vi "Initialize-user-events.vi"(8 "error in (no error)":errorcluster, 11 "Object ref in":T1) -> (0 "error out":errorcluster, 3 "Object ref out":T1)   [LabVIEW 2013, in "HardwareCharacterization.lvlib" / "HC-Main.lvclass"]
uses:
  HC-Main.lvclass
  Object-reference.ctl
  HC-Main.lvclass/HC-Main.ctl
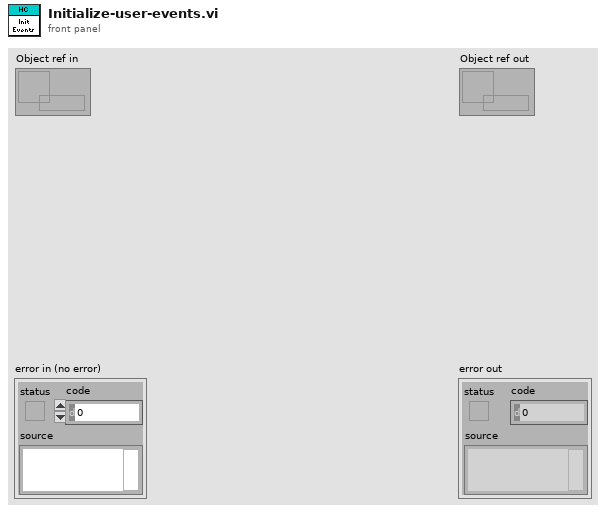
[diagram p1: front panel]
types:
  T1 = typedef "HardwareCharacterization.lvlib/HC-Main.lvclass/Object-reference.ctl" = refnum<data-value>
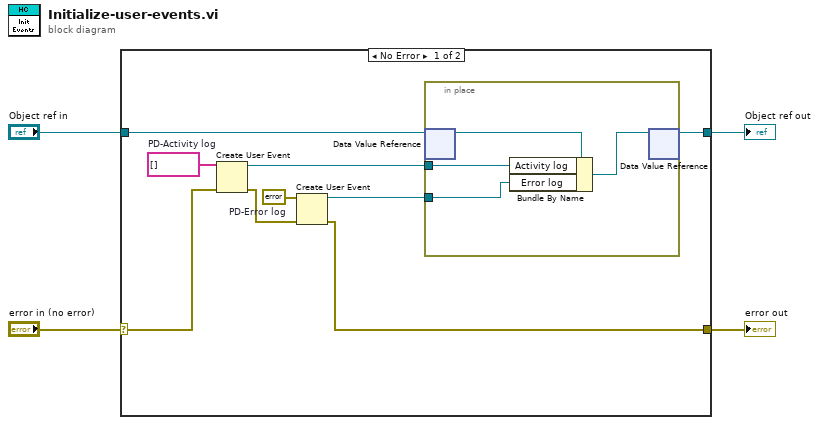
[diagram p0: block diagram]
diagram:
  n1 = case shown="No Error" "error in (no error)" {
    selector: "error in (no error)" -> [w9 w19]
    tunnel: [w10 w19] -> w3
    tunnel: [w12 w18] -> w1
    tunnel: "Object ref in" -> [w13 w18]
    frame No Error {
      w5 = string[] []  # PD-Activity log
      w8 = errorcluster {"status"=FALSE, "code"=0, "source"=""}  # PD-Error log
      n2 = Create User Event(user event datatype=w5, error in=w9) -> (user event=w7:refnum<user-event>, error out=w11:errorcluster)
      n3 = Create User Event(user event datatype=w8, error in=w11) -> (user event=w6:refnum<user-event>, error out=w10:errorcluster)
      n4 = in-place {
        in-place-border: w7 -> [w14]
        in-place-border: w6 -> [w15]
        n5 = in-place-dvr #1(w13) -> (w17:refnum<class "HC-Main.lvclass">)  [unwired: 1 out]
        n6 = Bundle By Name(cluster=w17, "Activity log"=w14, "Error log"=w15) -> (w16:refnum<class "HC-Main.lvclass">)
        n7 = in-place-dvr #1(w16) -> (w12:T1)  [unwired: 1 out]
      }
    }
    frame Error {
    }
  }
  "error out" <- w3
  "Object ref out" <- w1
